vi "PH_Stepmotor_BaseClass.set GUI Refs.vi"(0 "i ref in":refnum<vi>, 1 "Class":string, 2 "GUI Refs":T2, 5 "error in":errorcluster) -> (14 "i ref out":refnum<vi>, 19 "error out":errorcluster)   [LabVIEW 2014, in "PH_Stepmotor_BaseClass.lvlib"]
doc: "This VI is forseen to set the GUI element references; it shall be used especially within child classes."
uses:
  PH_Stepmotor_BaseClass.lvlib
  PH_Stepmotor_BaseClass.GUI Refs.ctl
  PH_Common/PH_Common.lvlib
  PH_PSDBWriter/PH_PSDBWriter.lvlib
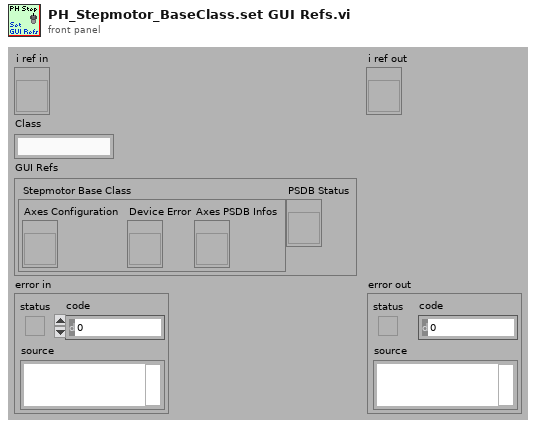
[diagram p1: front panel]
types:
  T1 = typedef "PH_Stepmotor_BaseClass.lvlib/PH_Stepmotor_BaseClass.GUI Refs.ctl" = cluster{"Axes Configuration":refnum<vi>, "Device Error":refnum<vi>, "Axes PSDB Infos":refnum<vi>}
  T2 = cluster{"Stepmotor Base Class ":T1, "PSDB Status":refnum<vi>}
  T3 = typedef "PH_Stepmotor_BaseClass.lvlib/PH_Stepmotor_BaseClass.i attribute.ctl" = cluster{"Device Error":errorcluster, "Axes PSDB Thread":cluster{"Ref":refnum<vi>, "Q-Ref":refnum<queue>, "Data Status":T4}, "Axes":T5[], "Axes PSDB Infos":cluster{"GUI Name":string, "PSDB Instance ID":i32, "PSDB Status Service ID":i32, "Axis":i32, "Class":string}[], "GUI Refs":T1}
  T4 = typedef "PH_PSDBWriter.lvlib/PH_PSDBWriter.Data Status.ctl" = i16
  T5 = typedef "PH_Stepmotor_BaseClass.lvlib/PH_Stepmotor_BaseClass.Axis Attributes.ctl" = cluster{"Settings":T6, "Endswitch?":bool, "DIM Service IDs":T8, "Activity":T9, "Configured?":bool, "Position":cluster{"Current":i32, "Target":i32}, "Position to set":cluster{"New?":bool, "Wanted":i32}, "Stop?":bool, "Reset?":bool, "Move?":bool, "Nothing connected?":bool}
  T6 = typedef "PH_Stepmotor_BaseClass.lvlib/PH_Stepmotor_BaseClass.Axis Settings.ctl" = cluster{"Sign change":bool, "Width":dbl, "Calibration":dbl, "Unit":string, "Motor Type":T7, "Unit Width":string, "Unit CF":string}
  T7 = typedef "PH_Stepmotor_BaseClass.lvlib/PH_Stepmotor_BaseClass.Motor Type.ctl" = enum16{"Unspecific", "OWIS 49.120.2633", "OWIS 49.060.1033", "OWIS 43.040.2558", "Diamond Motion 2200 series", "OWIS 49.120.266B.MV6", "Calorimeter", "Linear Stage 1", "MICOS VT-80", "MICOS VT-80 S", "Standa Rotstage nt0.95A", "PUF RA 320.200", "PUF RA 800.200", "PUF RA 800.400", "PUF RA 400.50", "1324.nn.800.50", "1324.n9c.800.50", "1324.nn.320.200", "1324.nn.400.200", "1324.nn.800.200", "1324.nn.400.50", "1324.8c9c.800.50", "1324.8c9c.400.200"}
  T8 = typedef "PH_Stepmotor_BaseClass.lvlib/PH_Stepmotor_BaseClass.Axis DIM Service IDs.ctl" = cluster{"Settings":i32, "Information":i32}
  T9 = typedef "PH_Stepmotor_BaseClass.lvlib/PH_Stepmotor_BaseClass.Axis Activity.ctl" = enum16{"No Information", "stopped", "running", "Failure", "Alarm", "stopped at backward ES", "stopped at foreward ES"}
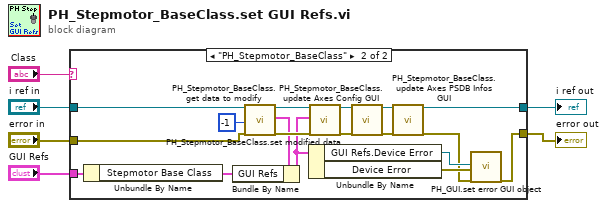
[diagram p0: block diagram]
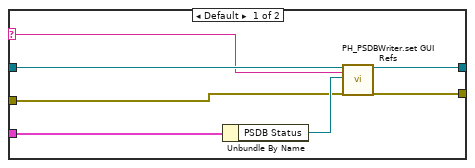
[diagram p2: hidden frame]
diagram:
  n1 = case shown="\"PH_Stepmotor_BaseClass\"" "Class" {
    selector: "Class" -> [w10 _]
    tunnel: "error in" -> [w8 w31]
    tunnel: "i ref in" -> [w11 w30]
    tunnel: [w7 w14] -> w4
    tunnel: [w9 w15] -> w3
    tunnel: "GUI Refs" -> [w12 w17]
    frame Default {
      n2 = Unbundle By Name(w12) -> ("PSDB Status"=w13:refnum<vi>)
      n3 = call "PH_PSDBWriter.set GUI Refs.vi"("i ref in"=w11, "Class"=w10, "Ref PSDB Status"=w13, "error in"=w8) -> ("i ref out"=w9:refnum<vi>, "error out"=w7:errorcluster)  [unwired: 14 in]
    }
    frame "PH_Stepmotor_BaseClass" {
      n4 = Unbundle By Name(w17) -> ("Stepmotor Base Class"=w16:T1)
      n5 = call "PH_Stepmotor_BaseClass.get data to modify.vi"("i ref in"=w30, "ms timeout (10000)"=-1, "error in (no error)"=w31) -> ("i ref out"=w27:refnum<vi>, "i attribute"=w26:T3, "error out"=w28:errorcluster)  [unwired: 13 in, 1 out]
      n6 = Bundle By Name(cluster=w26, "GUI Refs"=w16) -> (w22:T3)
      n7 = Unbundle By Name(w22) -> ("GUI Refs.Device Error"=w20:refnum<vi>, "Device Error"=w21:errorcluster)
      n8 = call "PH_Stepmotor_BaseClass.set modified data.vi"("i ref in"=w27, "i attribute"=w22, "error in (no error)"=w28) -> ("i ref out"=w25:refnum<vi>, "error out"=w24:errorcluster)  [unwired: 15 in]
      n9 = call "PH_Stepmotor_BaseClass.update Axes Config GUI.vi"("VI in"=w25, "error in (no error)"=w24) -> ("VI out"=w18:refnum<vi>, "error out"=w23:errorcluster)  [unwired: 16 in]
      n10 = call "PH_Stepmotor_BaseClass.update Axes PSDB Infos GUI.vi"("VI in"=w18, "error in (no error)"=w23) -> ("VI out"=w15:refnum<vi>, "error out"=w19:errorcluster)  [unwired: 16 in]
      n11 = call "PH_GUI.set error GUI object.vi"("GUI Refs.Device Error"=w20, "error to set"=w21, "error in (no error)"=w19) -> ("error out"=w14:errorcluster)  [unwired: 16 in]
    }
  }
  "error out" <- w4
  "i ref out" <- w3
